vi "Clean Up.vi"(0 "Process Handler In":refnum<class "Process Handler.lvclass">, 1 "Timeout in ms (-1)":i32=-1, 11 "Error In":errorcluster) -> (4 "Process Handler Out":refnum<class "Process Handler.lvclass">, 15 "Error Out":errorcluster)   [LabVIEW 2023, in "Process Handler.lvclass"]
doc: "Stops all spawn processes and then itself."
uses:
  Process Handler.lvclass
  Interfaces/ICanCommunicate/Message.ctl
  Process Handler.lvclass/Process Handler.ctl
  Interfaces/ICanCommunicate/ICanCommunicate.lvclass
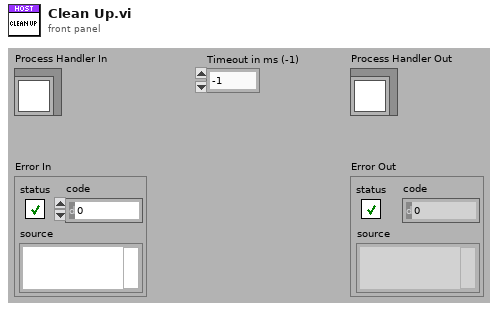
[diagram p1: front panel]
types:
  T1 = typedef "ICanCommunicate.lvclass/Message.ctl" = cluster{"Sender Name":string, "Recipent Name":string, "Command":string, "Data":variant, "Signature":string}
  T2 = enum16{"ReadRepository", "CreateNew", "CreateOrLookUpExisting", "ReadRepositoryAndDestroy"}
  T3 = typedef "ICanCommunicate.lvclass/ProcessSyncQueue.ctl" = refnum<queue>
  T4 = typedef "ICanCommunicate.lvclass/FromProcessQueue.ctl" = refnum<queue>
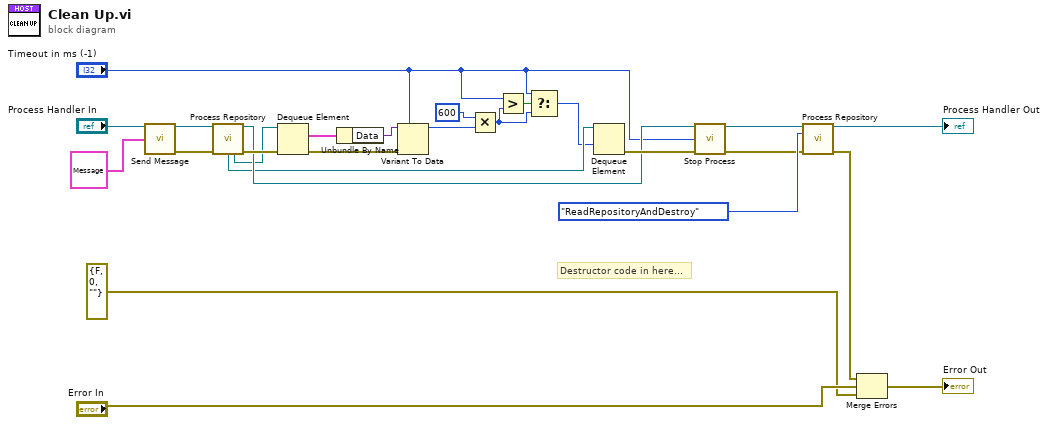
[diagram p0: block diagram]
diagram:
  # "Destructor code in here..."
  n1 = call-dynamic "Send Message.vi"("ICanCommunicate In"="Process Handler In", "Message"=T1 {"Sender Name"="", "Recipent Name"="", "Command"="End Spawn Processes", "Data"=variant, "Signature"=""}) -> ("ICanCommunicate Out"=w13:refnum<class "Process Handler.lvclass">, "Error Out"=w17:errorcluster)  [unwired: 12 in]
  n2 = call-dynamic "Process Repository.vi"("Process In"=w13, "Error In"=w17) -> ("Process Out"=w12:refnum<class "Process Handler.lvclass">, "ProcessSyncQueue"=w11:T3, "FromProcessQueue"=w10:T4, "Error Out"=w14:errorcluster)  [unwired: 7 in, 3 out]
  n3 = Dequeue Element(queue=w10, error in (no error)=w14) -> (element=w9:T1, error out=w7:errorcluster)  [unwired: 1 in, 2 out]
  n4 = Unbundle By Name(w9) -> ("Data"=w8:variant)
  n5 = Variant To Data(error in=w7, type="Timeout in ms (-1)", Variant=w8) -> (data=w6:i32)  [unwired: 1 out]
  n6 = Multiply(x=600, y=w6) -> (x*y=w3:i32)
  n7 = Greater?(x="Timeout in ms (-1)", y=w3) -> (0:w4:bool)
  n8 = Select(t="Timeout in ms (-1)", s=w4, f=w3) -> (s? t:f=w2:i32)
  n9 = Dequeue Element(queue=w11, timeout in ms (-1)=w2) -> (error out=w15:errorcluster)  [unwired: 1 in, 3 out]
  n10 = call-dynamic "Stop Process.vi"("Process In"=w12, "Timeout in ms (-1)"="Timeout in ms (-1)", "Error In"=w15) -> ("Process Out"=w25:refnum<class "Process Handler.lvclass">, "Error Out"=w23:errorcluster)  [unwired: 11 in]
  n11 = call-dynamic "Process Repository.vi"("Process In"=w25, "Action(ReadRepository)"=T2."ReadRepositoryAndDestroy", "Error In"=w23) -> ("Process Out"=→"Process Handler Out":refnum<class "Process Handler.lvclass">, "Error Out"=w24:errorcluster)  [unwired: 6 in, 5 out]
  n12 = Merge Errors(w24, "Error In", errorcluster {"status"=FALSE, "code"=0, "source"=""} ("error in (no error)")) -> (→"Error Out":errorcluster)
